vi "Rinocloud_HTTP_ancestors.vi"(4 "error in (no error)":errorcluster, 7 "id":string) -> (0 "error out":errorcluster, 1 "Status":T2={"headers"="", "body"="", "ID"="", "Saved"=TRUE}, 2 "last ID":string, 3 "metadata array":T1(array[cluster]))   [LabVIEW 2011, in "Rinocloud Library.lvlib"]
uses:
  Rinocloud Library.lvlib
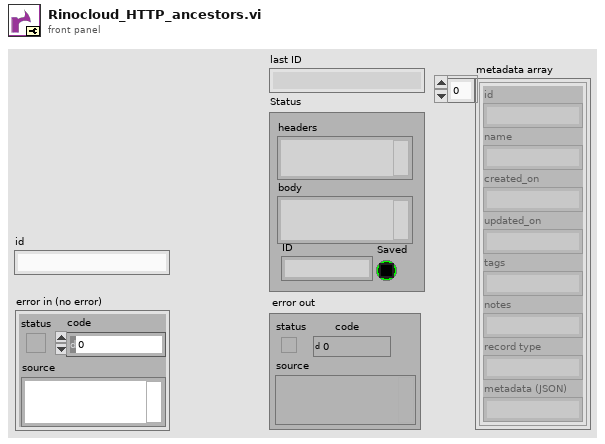
[diagram p1: front panel]
types:
  T1 = cluster{"id":string, "name":string, "created_on":string, "updated_on":string, "tags":string, "notes":string, "record type":string, "metadata (JSON)":string}[]
  T2 = cluster{"headers":string, "body":string, "ID":string, "Saved":bool}
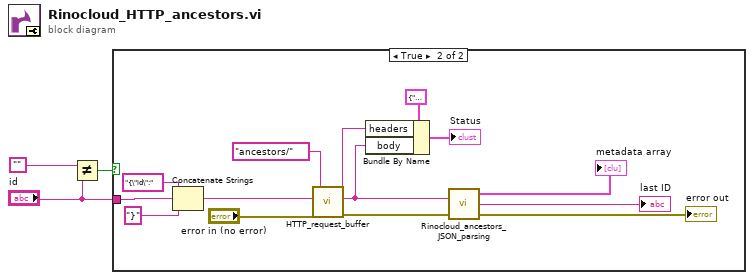
[diagram p0: block diagram]
diagram:
  n1 = Not Equal?(x="", y="id") -> (x != y?=w1:bool)
  n2 = case shown="True" w1 {
    tunnel: "id" -> [_ w5]
    frame False {
    }
    frame True {
      n3 = Concatenate Strings("{\"id\":" ("string"), w5, "}" ("string")) -> (w4:string)
      n4 = call "HTTP_request_buffer.vi"("error in (no error)"="error in (no error)", "JSON payload"=w4, "Endpoint"="ancestors/") -> ("error out"=w16:errorcluster, "body"=w17:string, "headers"=w15:string)  [unwired: 2 in]
      n5 = Bundle By Name(cluster=T2 {"headers"="", "body"="", "ID"="", "Saved"=TRUE} ("Status 2"), "headers"=w15, "body"=w17) -> (→"Status":T2)
      n6 = call "Rinocloud_ancestors_JSON_parsing.vi"("error in (no error)"=w16, "JSON string"=w17) -> ("error out"=→"error out":errorcluster, "last ID"=→"last ID":string, "metadata array"=→"metadata array":T1)  [unwired: 1 in]
    }
  }
